vi "HapticSTM-Demod.vi"() -> ()   [LabVIEW 2019]
uses:
  <userlib>/HapticSTM/HapticSTM.lvlib
panel:
  in  "Signal":u16(ring) items=["Z Val", "Demod"]
  in  "Save":bool
  out "Origin Y":dbl
  out "Origin X":dbl
  out "Arm output":dbl
  in  "Rough adjust":dbl
  out "ZVAL":dbl
  out "Y Out":dbl
  out "X Out":dbl
  out "Max speed":dbl
  out "Width":dbl
  out "VY":dbl
  out "VZ":dbl
  out "VX":dbl
  in  "Drag":dbl=1.0
  in  "STOP":bool
  in  "START":bool
  out "Fy":dbl
  out "Fz":dbl
  out "phi":dbl
  out "psi":dbl
  out "Fx":dbl
  out "theta":dbl
  out "x":dbl
  out "y":dbl
  out "z":dbl
  in  "Fine adjust":dbl=3.5
  out "Clicks":dbl
  out "Height":dbl
  # "Sample Window"
  # "Position"
  # "Sensitivity"
  # "Force"
  # "STM I/O"
  # "Angles"
  # "Velocity"
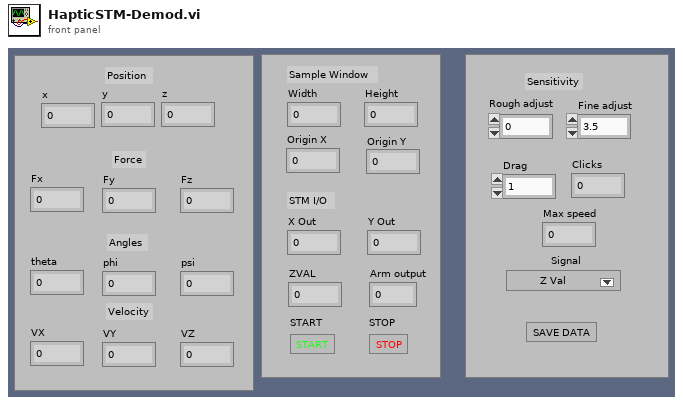
[diagram p1: front panel]
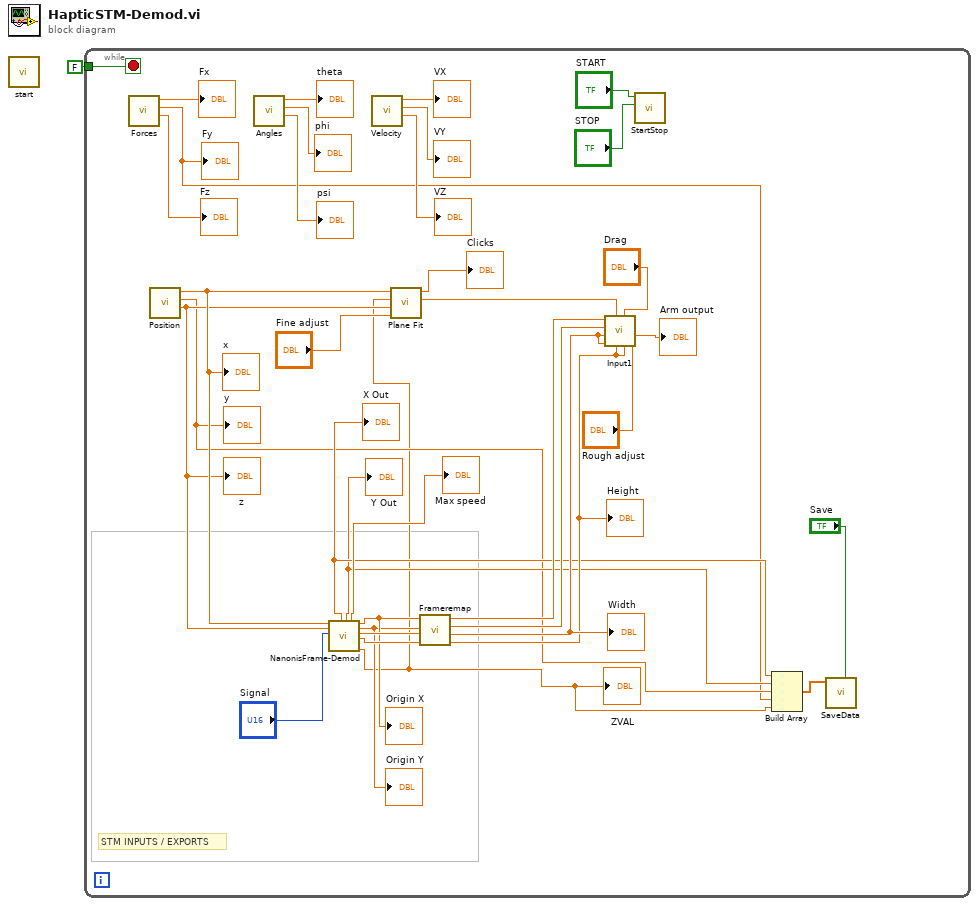
[diagram p0: block diagram]
diagram:
  n1 = call <userlib>:"start.vi"() -> ()  [unwired: 11 in, 1 out]
  n2 = while {
    tunnel: FALSE -> [w27]
    stop <- w27 stop-if-true
    # "STM INPUTS / EXPORTS"
    n3 = call "Forces.vi"() -> ("Fz"=→"Fz":dbl, "Fy"=w6:dbl, "Fx"=→"Fx":dbl)  [unwired: 9 in]
    "Fy" <- w6
    n4 = call "Position.vi"() -> ("Z"=w17:dbl, "Y"=w7:dbl, "X"=w18:dbl)  [unwired: 9 in]
    "x" <- w18
    "y" <- w7
    "z" <- w17
    n5 = call "Angles.vi"() -> ("psi"=→"psi":dbl, "phi"=→"phi":dbl, "theta"=→"theta":dbl)  [unwired: 9 in]
    n6 = call "NanonisFrame-Demod.vi"("x"=w18, "z"=w17, "Signal"="Signal") -> ("X Out"=w9:dbl, "Z Out"=w8:dbl, "Speed"=→"Max speed":dbl, "FO X"=w11:dbl, "FO Z"=w10:dbl, "FW"=w15:dbl, "FH"=w14:dbl, "CVAL (nA)"=w5:dbl)  [unwired: 9 in]
    "Y Out" <- w8
    "X Out" <- w9
    "ZVAL" <- w5
    "Origin X" <- w11
    "Origin Y" <- w10
    n7 = call "Velocity.vi"() -> ("VZ"=→"VZ":dbl, "VY"=→"VY":dbl, "VX"=→"VX":dbl)  [unwired: 9 in]
    n8 = call "Plane Fit.vi"("Sensitivity"="Fine adjust", "Z"=w17, "Nano Z"=w5, "X"=w18) -> ("Output"=w30:dbl, "Clicks"=→"Clicks":dbl)  [unwired: 6 in]
    n9 = call "Frameremap.vi"("FH"=w14, "FW"=w15, "FO Z"=w10, "FO X"=w11) -> ("FH"=w19:dbl, "FW"=w20:dbl, "Z Origin"=w28:dbl, "X Origin"=w29:dbl)  [unwired: 4 in]
    "Height" <- w19
    "Width" <- w20
    n10 = call "Input1.vi"("Current * 10^input"="Rough adjust", "Scopez"=w19, "Drag"="Drag", "FH"=w19, "Signal in"=w30, "FW"=w20, "Scopex"=w20, "Z origin"=w28, "X origin"=w29) -> ("Scaled Current"=→"Arm output":dbl)  [unwired: 2 in]
    n11 = call "StartStop.vi"("STOP"="STOP", "START"="START") -> ()  [unwired: 10 in]
    n12 = Build Array(w9, w8, w7, w6, w5) -> (w4:dbl[])
    n13 = call "SaveData.vi"("Save"="Save", "Data"=w4) -> ()  [unwired: 10 in]
  }
